vi "字节在前高字节在后.vi"(11 "数值输入":dbl) -> (2 "高字节":u16, 3 "低字节":u8)   [LabVIEW 2016]
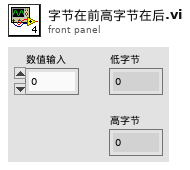
[diagram p1: front panel]
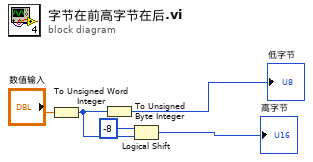
[diagram p0: block diagram]
diagram:
  n1 = To Unsigned Word Integer(number="数值输入") -> (unsigned 16bit integer=w5:u16)
  n2 = To Unsigned Byte Integer(number=w5) -> (unsigned 8bit integer=→"低字节":u8)
  n3 = Logical Shift(y=i16 -8, x=w5) -> (x << y=→"高字节":u16)
